vi "NormalizeArray.vi"(1 "Magnitude of Spectrun":cluster{"x0":dbl, "df":dbl, dbl[]}(graph)) -> (0 "Magnitude of Spectrun":cluster{"x0":dbl, "df":dbl, dbl[]}(graph))   [LabVIEW 2022 SP3]
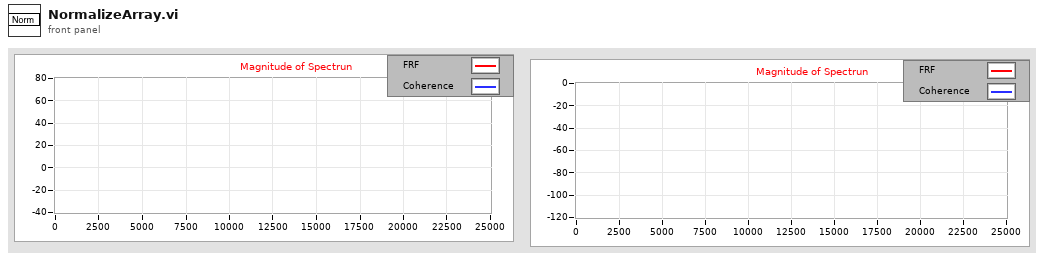
[diagram p1: front panel]
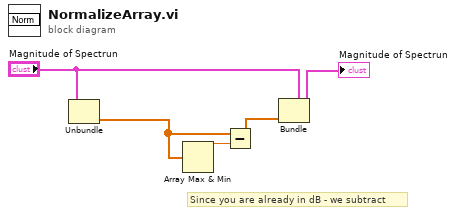
[diagram p0: block diagram]
diagram:
  # "Since you are already in dB - we subtract"
  n1 = Unbundle("Magnitude of Spectrun") -> (w4:dbl[])  [unwired: 2 out]
  n2 = Array Max & Min(array=w4) -> (max value=w5:dbl)  [unwired: 3 out]
  n3 = Subtract(x=w4, y=w5) -> (x-y=w2:dbl[])
  n4 = Bundle(cluster="Magnitude of Spectrun", w2) -> (→"Magnitude of Spectrun":cluster{"x0":dbl, "df":dbl, dbl[]})  [unwired: 2 in]
